vi "Autonomous Independent.vi"() -> ()   [LabVIEW 2014]
doc: "This VI is called when autonomous begins, and will automatically be terminated when autonomous ends. You can carry out timed or sensor driven robot movement independently without needing to return to the caller."
uses:
  Robot Global Data.vi
panel:
  in  "Numeric":i32
  # "Be sure to right-click and choose Data Operations>>Make Current Value default if you want to save the array values with the VI"
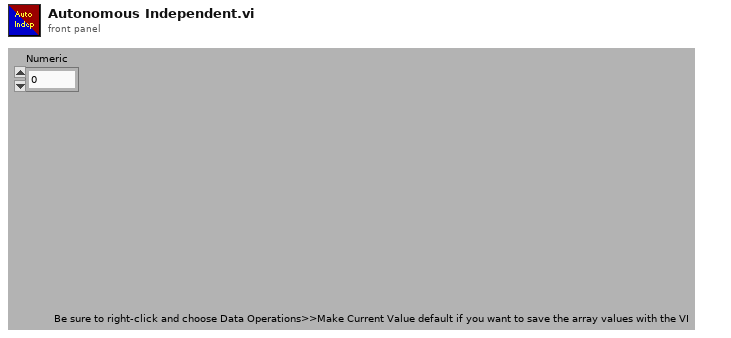
[diagram p1: front panel]
types:
  T1 = cluster{"Numeric":dbl, cluster{"Numeric out":dbl, "Numeric":dbl, dbl}, cluster{"Numeric":dbl, "Numeric":dbl, "upper limit":dbl, "Numeric":dbl, "Numeric":dbl, "upper limit":dbl}}
  T2 = cluster{"Numeric":dbl, "Numeric":dbl, "upper limit":dbl, "Numeric":dbl, "Numeric":dbl, "upper limit":dbl}
  T3 = cluster{"Numeric":dbl, cluster{dbl, dbl, dbl}, cluster{"Numeric":dbl, "Numeric":dbl, "upper limit":dbl, "Numeric":dbl, "Numeric":dbl, "upper limit":dbl}}
  T4 = cluster{"Numeric":dbl, cluster{"Numeric out":dbl, dbl, "Numeric":dbl}, cluster{"Numeric":dbl, "Numeric":dbl, "upper limit":dbl, "Numeric":dbl, "Numeric":dbl, "upper limit":dbl}}
  T5 = cluster{"Numeric":dbl, cluster{dbl, "Numeric out":dbl, "Numeric":dbl}, cluster{"Numeric":dbl, "Numeric":dbl, "upper limit":dbl, "Numeric":dbl, "Numeric":dbl, "upper limit":dbl}}
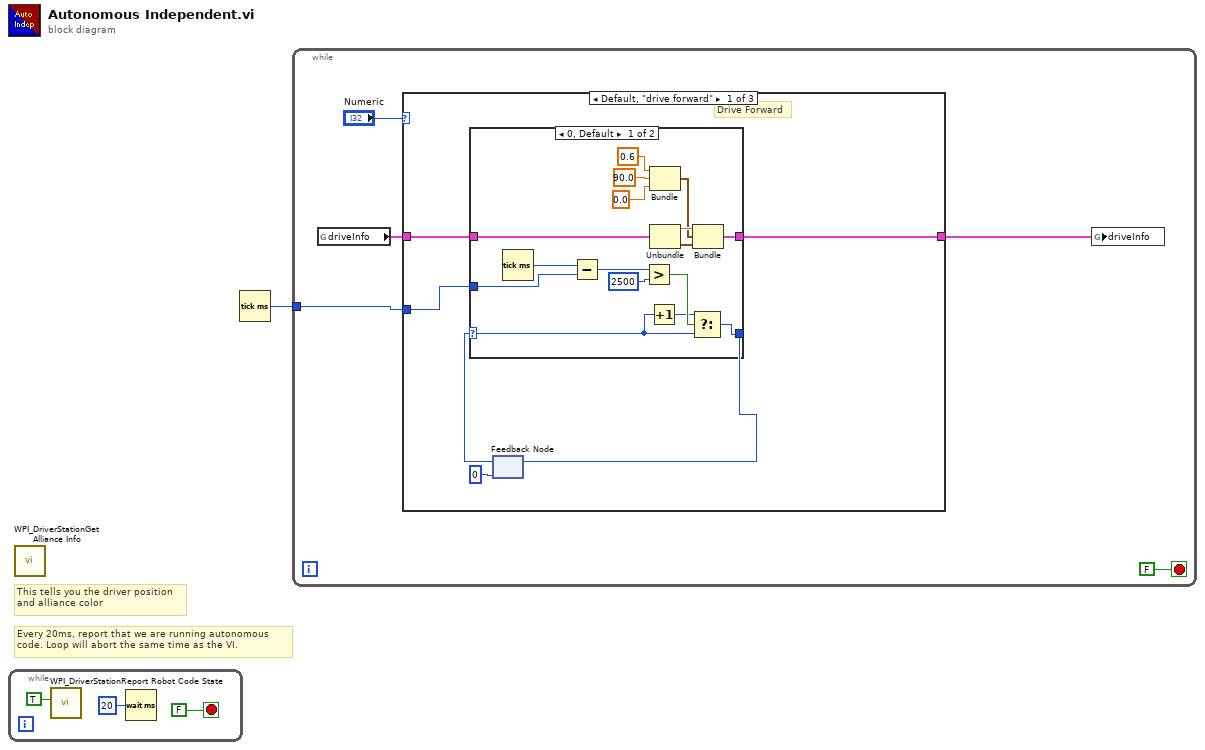
[diagram p0: block diagram]
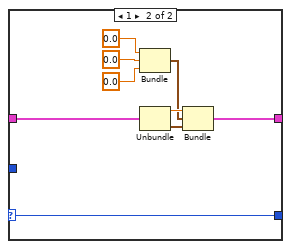
[diagram p2: hidden frame]
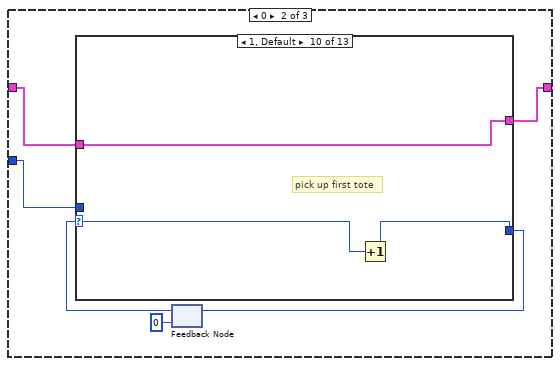
[diagram p3: hidden frame]
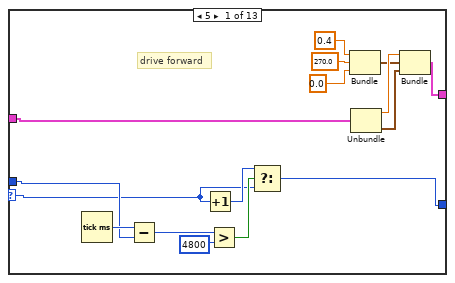
[diagram p4: hidden frame]
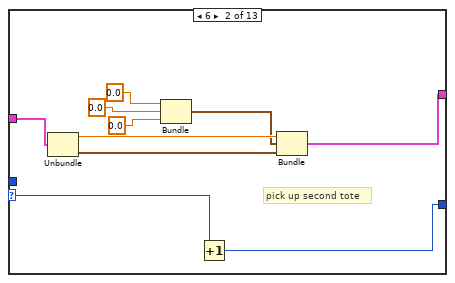
[diagram p5: hidden frame]
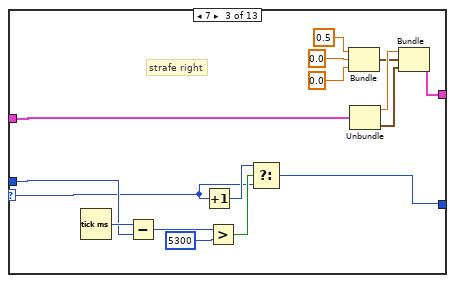
[diagram p6: hidden frame]
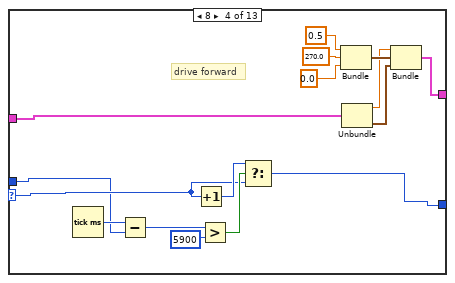
[diagram p7: hidden frame]
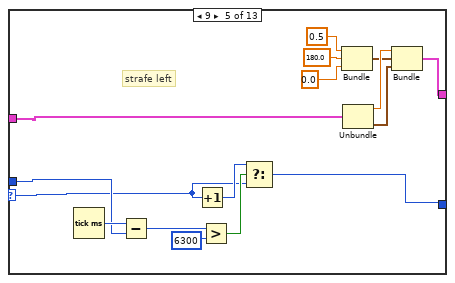
[diagram p8: hidden frame]
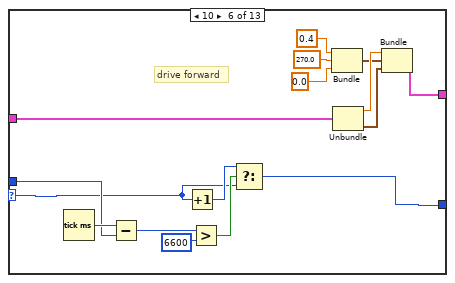
[diagram p9: hidden frame]
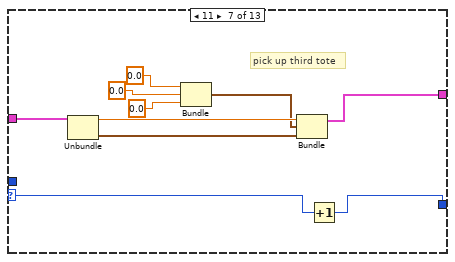
[diagram p10: hidden frame]
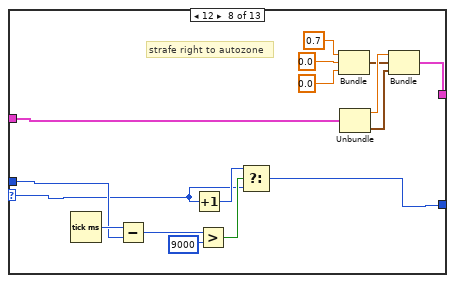
[diagram p11: hidden frame]
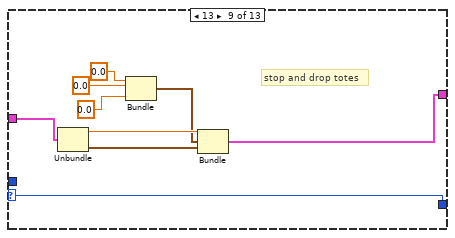
[diagram p12: hidden frame]
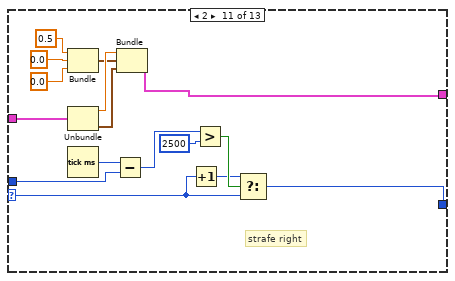
[diagram p13: hidden frame]
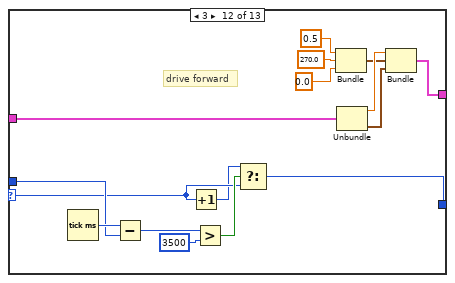
[diagram p14: hidden frame]
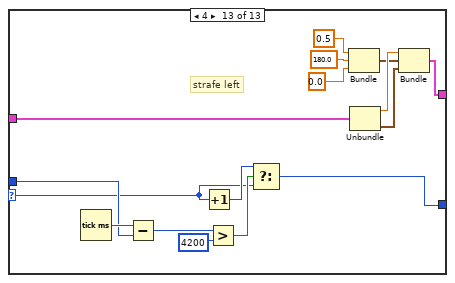
[diagram p15: hidden frame]
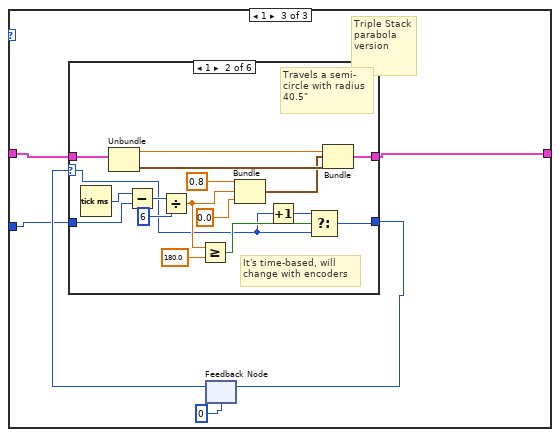
[diagram p16: hidden frame]
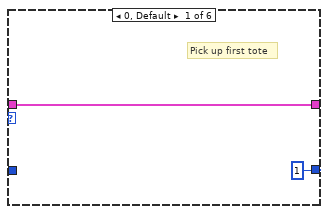
[diagram p17: hidden frame]
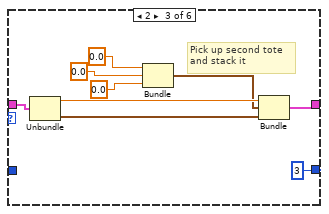
[diagram p18: hidden frame]
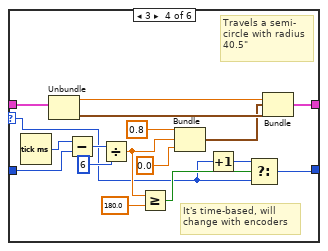
[diagram p19: hidden frame]
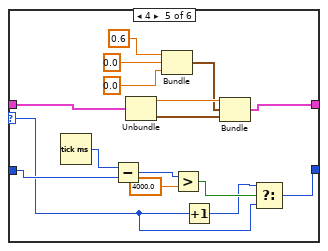
[diagram p20: hidden frame]
diagram:
  # "Every 20ms, report that we are running autonomous\ncode. Loop will abort the same time as the VI."
  # "This tells you the driver position\nand alliance color"
  n1 = while {
    stop <- FALSE stop-if-true
    n2 = call <vilib>:"WPI_DriverStationReport Robot Code State.vi"("Autonomous"=TRUE) -> ()  [unwired: 10 in, 1 out]
    n3 = Wait (ms)(milliseconds to wait=u32 20) -> ()  [unwired: 1 out]
  }
  n4 = call <vilib>:"WPI_DriverStationGet Alliance Info.vi"() -> ()  [unwired: 12 out]
  n5 = Tick Count (ms)() -> (millisecond timer value=w1:u32)
  n6 = while {
    tunnel: w1 -> [w6]
    stop <- FALSE stop-if-true
    n7 = global read "Robot Global Data.vi" "driveInfo"() -> (w8:T1)
    n8 = case shown="Default, \"drive forward\"" "Numeric" {
      tunnel: [w15 w42 w223] -> w7
      tunnel: w8 -> [w14 w46 w226]
      tunnel: w6 -> [w11 w45 w224]
      frame 2, Default {
        # "Drive Forward"
        n9 = feedback #1(0) -> (w12:i32)
        n10 = case shown="0, Default" w12 {
          selector: w12 -> [w20 w40]
          tunnel: [w31 w33] -> w15
          tunnel: w14 -> [w30 w34]
          tunnel: w11 -> [w16 _]
          tunnel: [w18 w40] -> w10
          frame 0, Default {
            n11 = Tick Count (ms)() -> (millisecond timer value=w17:u32)
            n12 = Subtract(x=w17, y=w16) -> (x-y=w23:u32)
            n13 = Greater?(x=w23, y=u32 2500) -> (0:w21:bool)
            n14 = Increment(x=w20) -> (x+1=w19:i32)
            n15 = Bundle(0.6, 90.0, 0.0) -> (w27:cluster{dbl, dbl, dbl})  [unwired: 1 in]
            n16 = Unbundle(w30) -> ("Numeric"=w29:dbl, w28:T2)  [unwired: 1 out]
            n17 = Select(t=w19, s=w21, f=w20) -> (s? t:f=w18:i32)
            n18 = Bundle("Numeric"=w29, w27, w28) -> (w31:T3)  [unwired: 1 in]
          }
          frame 1 {
            n19 = Bundle(0.0, 0.0, 0.0) -> (w37:cluster{dbl, dbl, dbl})  [unwired: 1 in]
            n20 = Unbundle(w34) -> ("Numeric"=w39:dbl, w38:T2)  [unwired: 1 out]
            n21 = Bundle("Numeric"=w39, w37, w38) -> (w33:T3)  [unwired: 1 in]
          }
        }
        n22 = feedback-in #1(w10) -> ()
      }
      frame 0 {
        n23 = feedback #2(u32 0 ("millisecond timer value")) -> (w44:u32)
        n24 = case shown="1, Default" w44 {
          selector: w44 -> [w51 w65 w76 w94 w108 w124 w139 w150 w163 w173 w177 w201 w211]
          tunnel: w46 -> [w50 w66 w78 w92 w110 w126 w140 w152 w165 w174 w190 w192 w209]
          tunnel: [w49 w63 w74 w91 w105 w122 w137 w148 w164 w174 w175 w191 w208] -> w42
          tunnel: w45 -> [w52 _ w77 w93 w109 w125 _ w151 _ _ w179 w205 w212]
          tunnel: [w48 w64 w75 w90 w107 w123 w138 w149 w163 w172 w176 w199 w210] -> w43
          frame 5 {
            # "drive forward"
            n25 = Tick Count (ms)() -> (millisecond timer value=w62:u32)
            n26 = Subtract(x=w62, y=w52) -> (x-y=w61:u32)
            n27 = Increment(x=w51) -> (x+1=w59:u32)
            n28 = Greater?(x=w61, y=u32 4800) -> (0:w60:bool)
            n29 = Select(t=w59, s=w60, f=w51) -> (s? t:f=w48:u32)
            n30 = Bundle(0.4, 270.0, 0.0) -> (w56:cluster{dbl, dbl, dbl})  [unwired: 1 in]
            n31 = Unbundle(w50) -> ("Numeric"=w58:dbl, w57:T2)  [unwired: 1 out]
            n32 = Bundle("Numeric"=w58, w56, w57) -> (w49:T3)  [unwired: 1 in]
          }
          frame 6 {
            # "pick up second tote"
            n33 = Unbundle(w66) -> ("Numeric"=w72:dbl, w71:T2)  [unwired: 1 out]
            n34 = Bundle(0.0, 0.0, 0.0) -> (w67:cluster{dbl, dbl, dbl})  [unwired: 1 in]
            n35 = Increment(x=w65) -> (x+1=w64:u32)
            n36 = Bundle("Numeric"=w72, w67, w71) -> (w63:T3)  [unwired: 1 in]
          }
          frame 7 {
            # "strafe right"
            n37 = Tick Count (ms)() -> (millisecond timer value=w88:u32)
            n38 = Subtract(x=w88, y=w77) -> (x-y=w87:u32)
            n39 = Increment(x=w76) -> (x+1=w85:u32)
            n40 = Greater?(x=w87, y=u32 5300) -> (0:w86:bool)
            n41 = Select(t=w85, s=w86, f=w76) -> (s? t:f=w75:u32)
            n42 = Bundle(0.5, 0.0, 0.0) -> (w82:cluster{dbl, dbl, dbl})  [unwired: 1 in]
            n43 = Unbundle(w78) -> ("Numeric"=w84:dbl, w83:T2)  [unwired: 1 out]
            n44 = Bundle("Numeric"=w84, w82, w83) -> (w74:T3)  [unwired: 1 in]
          }
          frame 8 {
            # "drive forward"
            n45 = Tick Count (ms)() -> (millisecond timer value=w95:u32)
            n46 = Subtract(x=w95, y=w93) -> (x-y=w96:u32)
            n47 = Increment(x=w94) -> (x+1=w98:u32)
            n48 = Greater?(x=w96, y=u32 5900) -> (0:w97:bool)
            n49 = Select(t=w98, s=w97, f=w94) -> (s? t:f=w90:u32)
            n50 = Bundle(0.5, 270.0, 0.0) -> (w101:cluster{dbl, dbl, dbl})  [unwired: 1 in]
            n51 = Unbundle(w92) -> ("Numeric"=w99:dbl, w100:T2)  [unwired: 1 out]
            n52 = Bundle("Numeric"=w99, w101, w100) -> (w91:T3)  [unwired: 1 in]
          }
          frame 9 {
            # "strafe left"
            n53 = Tick Count (ms)() -> (millisecond timer value=w120:u32)
            n54 = Subtract(x=w120, y=w109) -> (x-y=w119:u32)
            n55 = Increment(x=w108) -> (x+1=w117:u32)
            n56 = Greater?(x=w119, y=u32 6300) -> (0:w118:bool)
            n57 = Select(t=w117, s=w118, f=w108) -> (s? t:f=w107:u32)
            n58 = Bundle(0.5, 180.0, 0.0) -> (w114:cluster{dbl, dbl, dbl})  [unwired: 1 in]
            n59 = Unbundle(w110) -> ("Numeric"=w116:dbl, w115:T2)  [unwired: 1 out]
            n60 = Bundle("Numeric"=w116, w114, w115) -> (w105:T3)  [unwired: 1 in]
          }
          frame 10 {
            # "drive forward"
            n61 = Tick Count (ms)() -> (millisecond timer value=w136:u32)
            n62 = Subtract(x=w136, y=w125) -> (x-y=w135:u32)
            n63 = Increment(x=w124) -> (x+1=w133:u32)
            n64 = Greater?(x=w135, y=u32 6600) -> (0:w134:bool)
            n65 = Select(t=w133, s=w134, f=w124) -> (s? t:f=w123:u32)
            n66 = Bundle(0.4, 270.0, 0.0) -> (w130:cluster{dbl, dbl, dbl})  [unwired: 1 in]
            n67 = Unbundle(w126) -> ("Numeric"=w132:dbl, w131:T2)  [unwired: 1 out]
            n68 = Bundle("Numeric"=w132, w130, w131) -> (w122:T3)  [unwired: 1 in]
          }
          frame 11 {
            # "pick up third tote"
            n69 = Unbundle(w140) -> ("Numeric"=w146:dbl, w145:T2)  [unwired: 1 out]
            n70 = Bundle(0.0, 0.0, 0.0) -> (w141:cluster{dbl, dbl, dbl})  [unwired: 1 in]
            n71 = Bundle("Numeric"=w146, w141, w145) -> (w137:T3)  [unwired: 1 in]
            n72 = Increment(x=w139) -> (x+1=w138:u32)
          }
          frame 12 {
            # "strafe right to autozone"
            n73 = Tick Count (ms)() -> (millisecond timer value=w162:u32)
            n74 = Subtract(x=w162, y=w151) -> (x-y=w161:u32)
            n75 = Increment(x=w150) -> (x+1=w159:u32)
            n76 = Greater?(x=w161, y=u32 9000) -> (0:w160:bool)
            n77 = Select(t=w159, s=w160, f=w150) -> (s? t:f=w149:u32)
            n78 = Bundle(0.7, 0.0, 0.0) -> (w156:cluster{dbl, dbl, dbl})  [unwired: 1 in]
            n79 = Unbundle(w152) -> ("Numeric"=w158:dbl, w157:T2)  [unwired: 1 out]
            n80 = Bundle("Numeric"=w158, w156, w157) -> (w148:T3)  [unwired: 1 in]
          }
          frame 13 {
            # "stop and drop totes"
            n81 = Unbundle(w165) -> ("Numeric"=w168:dbl, w167:T2)  [unwired: 1 out]
            n82 = Bundle("Numeric out"=0.0, 0.0, "Numeric"=0.0) -> (w166:cluster{"Numeric out":dbl, dbl, "Numeric":dbl})  [unwired: 1 in]
            n83 = Bundle("Numeric"=w168, w166, w167) -> (w164:T4)  [unwired: 1 in]
          }
          frame 1, Default {
            # "pick up first tote"
            n84 = Increment(x=w173) -> (x+1=w172:u32)
          }
          frame 2 {
            # "strafe right"
            n85 = Bundle(0.5, 0.0, 0.0) -> (w187:cluster{dbl, dbl, dbl})  [unwired: 1 in]
            n86 = Unbundle(w190) -> ("Numeric"=w189:dbl, w188:T2)  [unwired: 1 out]
            n87 = Tick Count (ms)() -> (millisecond timer value=w183:u32)
            n88 = Subtract(x=w183, y=w179) -> (x-y=w182:u32)
            n89 = Bundle("Numeric"=w189, w187, w188) -> (w175:T3)  [unwired: 1 in]
            n90 = Increment(x=w177) -> (x+1=w178:u32)
            n91 = Greater?(x=w182, y=u32 2500) -> (0:w180:bool)
            n92 = Select(t=w178, s=w180, f=w177) -> (s? t:f=w176:u32)
          }
          frame 3 {
            # "drive forward"
            n93 = Tick Count (ms)() -> (millisecond timer value=w206:u32)
            n94 = Subtract(x=w206, y=w205) -> (x-y=w204:u32)
            n95 = Increment(x=w201) -> (x+1=w200:u32)
            n96 = Greater?(x=w204, y=u32 3500) -> (0:w202:bool)
            n97 = Select(t=w200, s=w202, f=w201) -> (s? t:f=w199:u32)
            n98 = Bundle(0.5, 270.0, 0.0) -> (w196:cluster{dbl, dbl, dbl})  [unwired: 1 in]
            n99 = Unbundle(w192) -> ("Numeric"=w198:dbl, w197:T2)  [unwired: 1 out]
            n100 = Bundle("Numeric"=w198, w196, w197) -> (w191:T3)  [unwired: 1 in]
          }
          frame 4 {
            # "strafe left"
            n101 = Tick Count (ms)() -> (millisecond timer value=w222:u32)
            n102 = Subtract(x=w222, y=w212) -> (x-y=w221:u32)
            n103 = Increment(x=w211) -> (x+1=w219:u32)
            n104 = Greater?(x=w221, y=u32 4200) -> (0:w220:bool)
            n105 = Select(t=w219, s=w220, f=w211) -> (s? t:f=w210:u32)
            n106 = Bundle(0.5, 180.0, 0.0) -> (w216:cluster{dbl, dbl, dbl})  [unwired: 1 in]
            n107 = Unbundle(w209) -> ("Numeric"=w218:dbl, w217:T2)  [unwired: 1 out]
            n108 = Bundle("Numeric"=w218, w216, w217) -> (w208:T3)  [unwired: 1 in]
          }
        }
        n109 = feedback-in #2(w43) -> ()
      }
      frame 1 {
        # "Triple Stack parabola version"
        n110 = feedback #3(0) -> (w227:i32)
        n111 = case shown="1" w227 {
          selector: w227 -> [_ w235 _ w261 w275 w290]
          tunnel: w226 -> [w229 w245 w255 w271 w289 w298]
          tunnel: [1 w233 3 w259 w274 w290] -> w225
          tunnel: w224 -> [_ w231 _ w257 w280 _]
          tunnel: [w229 w240 w252 w266 w282 w291] -> w223
          frame 0, Default {
            # "Pick up first tote"
          }
          frame 1 {
            # "It's time-based, will\nchange with encoders"
            # "Travels a semi-\ncircle with radius\n40.5\""
            n112 = Tick Count (ms)() -> (millisecond timer value=w232:u32)
            n113 = Unbundle(w245) -> ("Numeric"=w244:dbl, w243:T2)  [unwired: 1 out]
            n114 = Subtract(x=w232, y=w231) -> (x-y=w247:u32)
            n115 = Divide(x=w247, y=u32 6) -> (x/y=w238:dbl)
            n116 = Greater Or Equal?(x=w238, y=180.0) -> (x >= y?=w236:bool)
            n117 = Bundle(0.8, w238, 0.0) -> (w242:cluster{dbl, dbl, dbl})  [unwired: 1 in]
            n118 = Increment(x=w235) -> (x+1=w234:i32)
            n119 = Select(t=w234, s=w236, f=w235) -> (s? t:f=w233:i32)
            n120 = Bundle("Numeric"=w244, w242, w243) -> (w240:T3)  [unwired: 1 in]
          }
          frame 2 {
            # "Pick up second tote\nand stack it"
            n121 = Unbundle(w255) -> ("Numeric"=w254:dbl, w253:T2)  [unwired: 1 out]
            n122 = Bundle(0.0, 0.0, 0.0) -> (w248:cluster{dbl, dbl, dbl})  [unwired: 1 in]
            n123 = Bundle("Numeric"=w254, w248, w253) -> (w252:T3)  [unwired: 1 in]
          }
          frame 3 {
            # "It's time-based, will\nchange with encoders"
            # "Travels a semi-\ncircle with radius\n40.5\""
            n124 = Tick Count (ms)() -> (millisecond timer value=w258:u32)
            n125 = Unbundle(w271) -> ("Numeric"=w270:dbl, w269:T2)  [unwired: 1 out]
            n126 = Subtract(x=w258, y=w257) -> (x-y=w273:u32)
            n127 = Divide(x=w273, y=u32 6) -> (x/y=w264:dbl)
            n128 = Greater Or Equal?(x=w264, y=180.0) -> (x >= y?=w262:bool)
            n129 = Bundle(0.8, w264, 0.0) -> (w268:cluster{dbl, dbl, dbl})  [unwired: 1 in]
            n130 = Increment(x=w261) -> (x+1=w260:i32)
            n131 = Select(t=w260, s=w262, f=w261) -> (s? t:f=w259:i32)
            n132 = Bundle("Numeric"=w270, w268, w269) -> (w266:T3)  [unwired: 1 in]
          }
          frame 4 {
            n133 = Tick Count (ms)() -> (millisecond timer value=w281:u32)
            n134 = Subtract(x=w281, y=w280) -> (x-y=w278:u32)
            n135 = Unbundle(w289) -> ("Numeric"=w287:dbl, w288:T2)  [unwired: 1 out]
            n136 = Bundle(0.6, "Numeric out"=0.0, "Numeric"=0.0) -> (w283:cluster{dbl, "Numeric out":dbl, "Numeric":dbl})  [unwired: 1 in]
            n137 = Greater?(x=w278, y=4000.0) -> (0:w277:bool)
            n138 = Increment(x=w275) -> (x+1=w276:i32)
            n139 = Bundle("Numeric"=w287, w283, w288) -> (w282:T5)  [unwired: 1 in]
            n140 = Select(t=w276, s=w277, f=w275) -> (s? t:f=w274:i32)
          }
          frame 5 {
            # "Also drop the totes"
            n141 = Unbundle(w298) -> ("Numeric"=w294:dbl, w293:T2)  [unwired: 1 out]
            n142 = Bundle("Numeric out"=0.0, 0.0, "Numeric"=0.0) -> (w292:cluster{"Numeric out":dbl, dbl, "Numeric":dbl})  [unwired: 1 in]
            n143 = Bundle("Numeric"=w294, w292, w293) -> (w291:T4)  [unwired: 1 in]
          }
        }
        n144 = feedback-in #3(w225) -> ()
      }
    }
    n145 = global write "Robot Global Data.vi" "driveInfo"(w7) -> ()
  }
